vi "Auton Begin.vi"   [LabVIEW 2012]
uses:
  <vilib>/Rock Robotics/SystemInterfaces/DIO/FPGA_DIOChannel.ctl
  <vilib>/Rock Robotics/SystemInterfaces/Typedef/FPGA_TypedefDigitalModule.ctl
types:
  T1 = typedef "FPGA_DIOChannel.ctl" = enum8{"DIO 1", "DIO 2", "DIO 3", "DIO 4", "DIO 5", "DIO 6", "DIO 7", "DIO 8", "DIO 9", "DIO 10", "DIO 11", "DIO 12", "DIO 13", "DIO 14", "Invalid"}
  T2 = typedef "FPGA_TypedefDigitalModule.ctl" = enum16{"Digital Module 1", "Digital Module 2"}
  T3 = typedef "WPI_DigitalInputDevRef.ctl" = cluster{"DevStatus":errorcluster, "DIO Channel":T1, "Digital Module":T2}
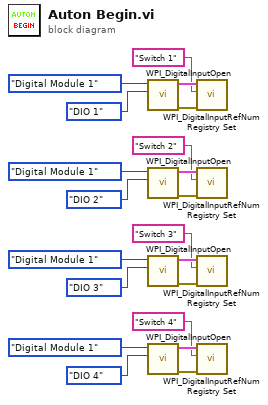
[diagram p0: block diagram]
diagram:
  n1 = call <vilib>:"WPI_DigitalInputOpen.vi"("DIO Channel"=FPGA_DIOChannel."DIO 1", "Digital Module (Module 1)"=FPGA_TypedefDigitalModule."Digital Module 1") -> ("error out"=w19:errorcluster, "DigitalInputDevRef"=w20:T3)  [unwired: 8 in]
  n2 = call <vilib>:"WPI_DigitalInputOpen.vi"("DIO Channel"=FPGA_DIOChannel."DIO 2", "Digital Module (Module 1)"=FPGA_TypedefDigitalModule."Digital Module 1") -> ("error out"=w14:errorcluster, "DigitalInputDevRef"=w13:T3)  [unwired: 8 in]
  n3 = call <vilib>:"WPI_DigitalInputOpen.vi"("DIO Channel"=FPGA_DIOChannel."DIO 3", "Digital Module (Module 1)"=FPGA_TypedefDigitalModule."Digital Module 1") -> ("error out"=w11:errorcluster, "DigitalInputDevRef"=w12:T3)  [unwired: 8 in]
  n4 = call <vilib>:"WPI_DigitalInputOpen.vi"("DIO Channel"=FPGA_DIOChannel."DIO 4", "Digital Module (Module 1)"=FPGA_TypedefDigitalModule."Digital Module 1") -> ("error out"=w6:errorcluster, "DigitalInputDevRef"=w5:T3)  [unwired: 8 in]
  n5 = call <vilib>:"WPI_DigitalInputRefNum Registry Set.vi"("error in (no error)"=w19, "refnum name"="Switch 1", "DigitalInputDevRef"=w20) -> ()  [unwired: 7 in, 2 out]
  n6 = call <vilib>:"WPI_DigitalInputRefNum Registry Set.vi"("error in (no error)"=w14, "refnum name"="Switch 2", "DigitalInputDevRef"=w13) -> ()  [unwired: 7 in, 2 out]
  n7 = call <vilib>:"WPI_DigitalInputRefNum Registry Set.vi"("error in (no error)"=w11, "refnum name"="Switch 3", "DigitalInputDevRef"=w12) -> ()  [unwired: 7 in, 2 out]
  n8 = call <vilib>:"WPI_DigitalInputRefNum Registry Set.vi"("error in (no error)"=w6, "refnum name"="Switch 4", "DigitalInputDevRef"=w5) -> ()  [unwired: 7 in, 2 out]
